vi "Construct Tx UDP.vi"(0 "custom device ref in":T6=18446744073709551615 format="%.0x", 1 "async loop rate hz":dbl, 5 "InstrumentHandle_board":u32, 7 "InstrumentHandle_port":u32, 9 "VL Configurations":T5(array[cluster]) {"VL Config"."NetSelect" items=["FDX_TX_FRAME_DLY_A"=0, "FDX_TX_FRAME_DLY_B"=1, "FDX_TX_FRAME_BOTH "=3, "FDX_TX_FRAME_ONLY_A"=4, "FDX_TX_FRAME_ONLY_B "=5]; "VL Config"."interfaceID" format="%.0b"}, 11 "error in (no error)":errorcluster, 12 "CommPort Payload":T2(array[cluster]) {"Parameters"."encoding" items=["BNR", "BCD", "Discrete", "Signed_32", "Signed_64", "Float_32", "Float_64", "Opaque"]}) -> (4 "custom device ref out":T6=18446744073709551615 format="%.0x", 6 "Execution Unit Out":refnum<class "Tx UDP Execution Unit.lvclass">, 15 "error out":errorcluster)   [LabVIEW 2020, in "AIM ARINC 664 Engine.lvlib" / "Implementation.lvlib" / "Tx UDP Execution Unit.lvclass"]
uses:
  Tx UDP Execution Unit.lvclass
  Execution Unit/Execution Unit.lvclass
  Execution Unit Factory/Execution Unit Factory.lvclass
  <vilib>/NI VeriStand/Custom Device API/Custom Device Item Ref.ctl
  <vilib>/NI VeriStand/Custom Device API/Custom Device API.lvlib
  Program Files/National Instruments/LabVIEW 2024/instr.lib/AIM GmbH/_AIM 664/_controls/comm_config_vl_tx.ctl
  Program Files/National Instruments/LabVIEW 2024/instr.lib/AIM GmbH/_AIM 664/AIM664LV.lvlib
  Program Files/National Instruments/LabVIEW 2024/instr.lib/AIM GmbH/_AIM 664/_controls/comm_udp_tx.ctl
  Shared/Encoding (Arinc664).ctl
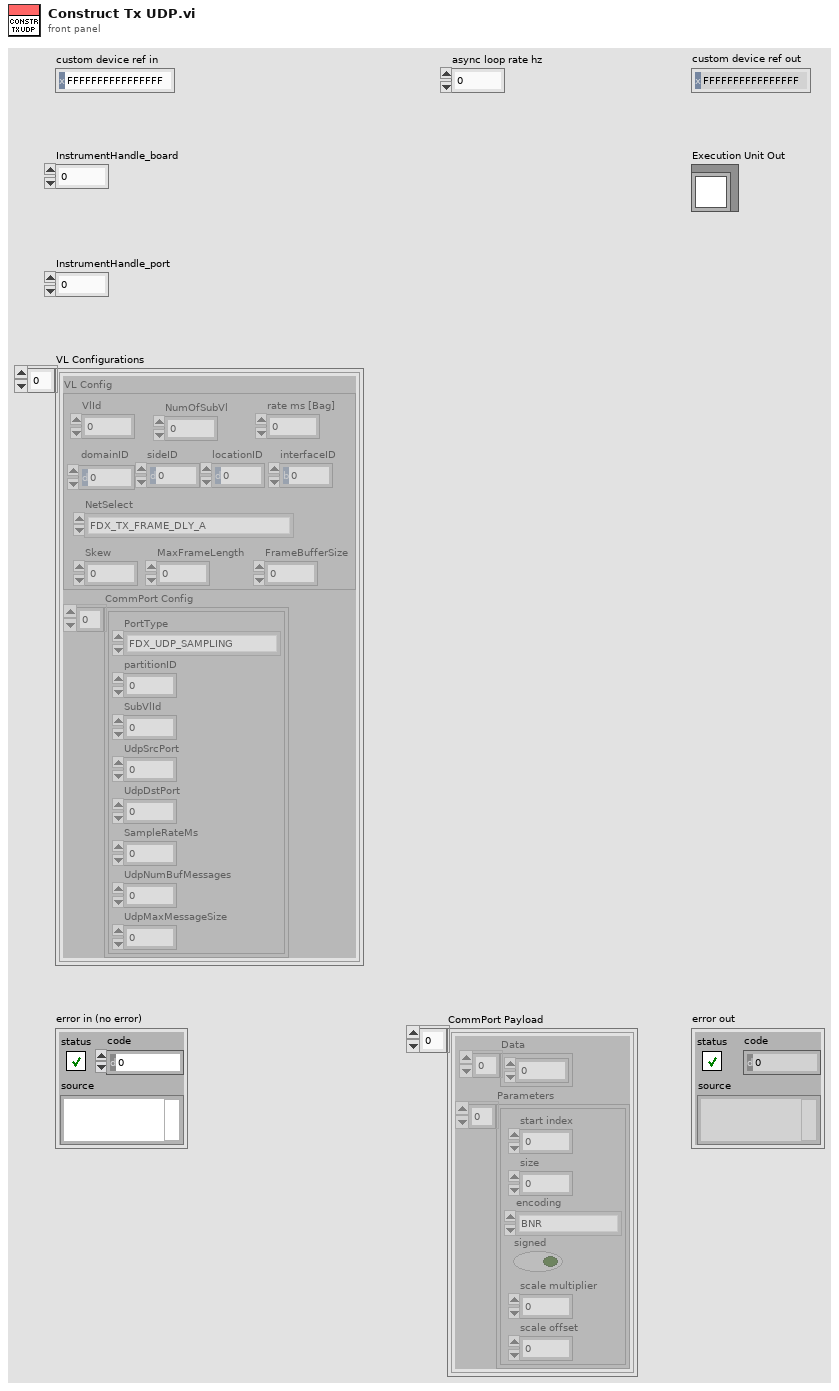
[diagram p1: front panel]
types:
  T1 = typedef "Encoding (Arinc664).ctl" = u16
  T2 = cluster{"Data":u8[], "Parameters":cluster{"start index":i32, "size":i32, "encoding":T1, "signed":bool, "scale multiplier":dbl, "scale offset":dbl}[]}[]
  T3 = typedef "AIM664LV.lvlib/comm_config_vl_tx.ctl" = cluster{"VlId":u16, "NumOfSubVl":u16, "rate ms [Bag]":u32, "domainID":u8, "sideID":u8, "locationID":u8, "interfaceID":u8, "NetSelect":u32, "Skew":u32, "MaxFrameLength":u32, "FrameBufferSize":u32}
  T4 = typedef "AIM664LV.lvlib/comm_udp_tx.ctl" = cluster{"PortType":enum16{"FDX_UDP_SAMPLING", "FDX_UDP_QUEUING"}, "partitionID":u8, "SubVlId":u8, "UdpSrcPort":u16, "UdpDstPort":u16, "SampleRateMs":dbl, "UdpNumBufMessages":u32, "UdpMaxMessageSize":u32}
  T5 = cluster{"VL Config":T3, "CommPort Config":T4[]}[]
  T6 = typedef "Custom Device API.lvlib/Custom Device Item Ref.ctl" = u64
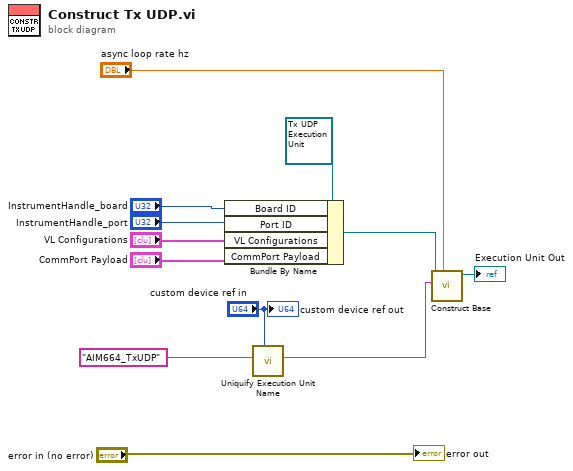
[diagram p0: block diagram]
diagram:
  n1 = Bundle By Name(cluster=refnum<class "Tx UDP Execution Unit.lvclass"> refnum ("Communication Bus Template Interfaces:Implementation.lvlib:Tx UDP Execution Unit.lvclass"), "Board ID"="InstrumentHandle_board", "Port ID"="InstrumentHandle_port", "VL Configurations"="VL Configurations", "CommPort Payload"="CommPort Payload") -> (w12:refnum<class "Tx UDP Execution Unit.lvclass">)
  n2 = call "Uniquify Execution Unit Name.vi"("custom device ref"="custom device ref in", "execution unit name"="AIM664_TxUDP") -> ("execution unit name out"=w10:string)  [unwired: 9 in]
  n3 = call "Construct Base.vi"("Execution Unit Implementation (default object)"=w12, "identifier"=w10, "async loop rate hz"="async loop rate hz") -> ("Execution Unit Out"=→"Execution Unit Out":refnum<class "Tx UDP Execution Unit.lvclass">)  [unwired: 6 in, 1 out]
  "error out" <- "error in (no error)"
  "custom device ref out" <- "custom device ref in"
